vi "Histogram Main.vi"() -> ()   [LabVIEW 2014]
uses:
  Consumer Message.ctl
panel:
  out "Waveform Chart":dbl[](graph)=[-0.7333632170503996, -1.4459924395536827, -0.6158814268082136, -1.631675160365316, -1.608798951635636, -1.2625195714755832, -1.4388813392251412, -2.3171612936361585, -2.012658397448811, -2.452817845479024, -1.872742142198202, -1.8081370028145534, -2.789563597879967, -1.8027089686061069, -2.322157895514915, -2.6951322450543405, -2.70911241695026, -1.9297374709836919, -2.579302146161715, -2.341637191084045, -2.916687331127644, -2.8232178479366854, -2.1046997729908883, -2.788310680238794, -2.64060281585839, -2.904801503797829, -2.083598772555009, -2.2414412347815467, -2.3134391852883973, -2.2472652262621815, -2.459431080647101, -1.5756227831916778, -1.7057574382014546, -1.0977978414739988, -1.595566141630414, -1.0423098355592761, -1.5626121000032929, -0.9136565974827924, -1.1678232599898863, -1.0064070705532606, -0.34750263923649743, -0.46884042157229494, 0.0019576712199835256, -0.25029780993618395, 0.4362619199660559, 0.23147283969027768, 0.7382142888428814, 0.6139801858185563, 1.0184032107197016, 0.7597297806877022, 1.4420680686425897, 1.1325435146385732, 1.720696415405159, 1.2439523984726168, 1.7812438958662287, 1.4653663148145577, 2.2007124336943167, 1.8367478777079433, 1.5463773683452176, 2.5440750285679083, 2.354209943920518, 2.504065470614749, 1.6572648013533686, 2.746716411146539, 2.4693516941541107, 2.0377544919327506, 2.028659531799731, 2.373684202132056, 2.030316257851516, 1.9944781194585937, 3.0612841364650025, 2.459440160574936, 2.695378131255343, 1.88317869797155, 2.4020213090840583, 1.9296628462729055, 2.0296568601608906, 2.662724277929503, 2.3134823505056046, 1.9158567122932988, 2.1398584968764776, 1.540815181341315, 1.3225488335799052, 1.7322571649762133, 1.449096031199046, 1.1359472555523311, 0.7462838155083935, 1.4330296047378257, 1.3257675163227414, 0.7403863574684398, 0.8139573928818378, 0.4596137579857783, 0.1374905254078728, -0.32650307170817594, -0.005885944408503383, -0.3876385007753408, 0.17942583515161425, -0.7655530391627472, -0.2667260819539556, -0.5640795763406656]
  in  "Snapshot":bool
  out "Histogram":cluster{"histogram":dbl[], "x axis":dbl[]}(graph)
  out "Consumer Shutdown?":bool=TRUE
  in  "Stop":bool
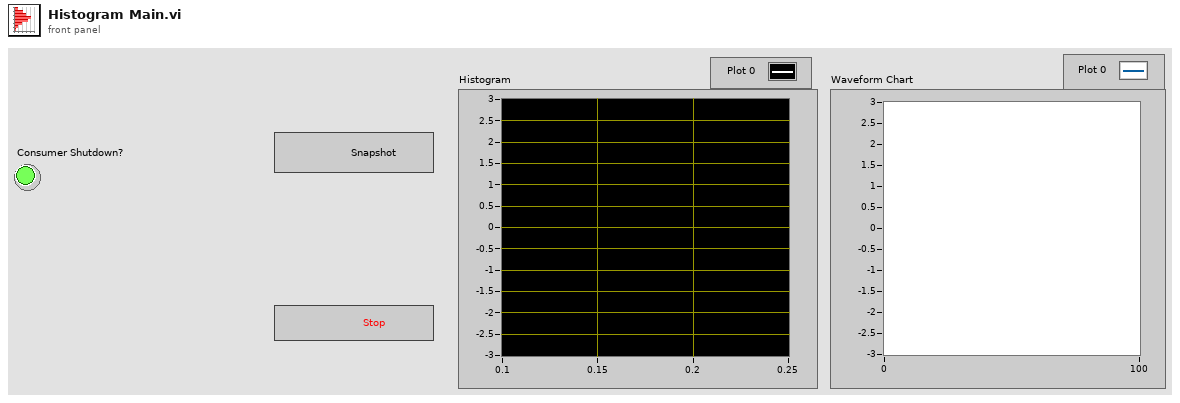
[diagram p1: front panel]
types:
  T1 = typedef "Consumer Message.ctl" = cluster{"Consumer State":string, "Boolean Data":bool, "Numeric Data":i32, "Signal":dbl[], "Error":errorcluster}
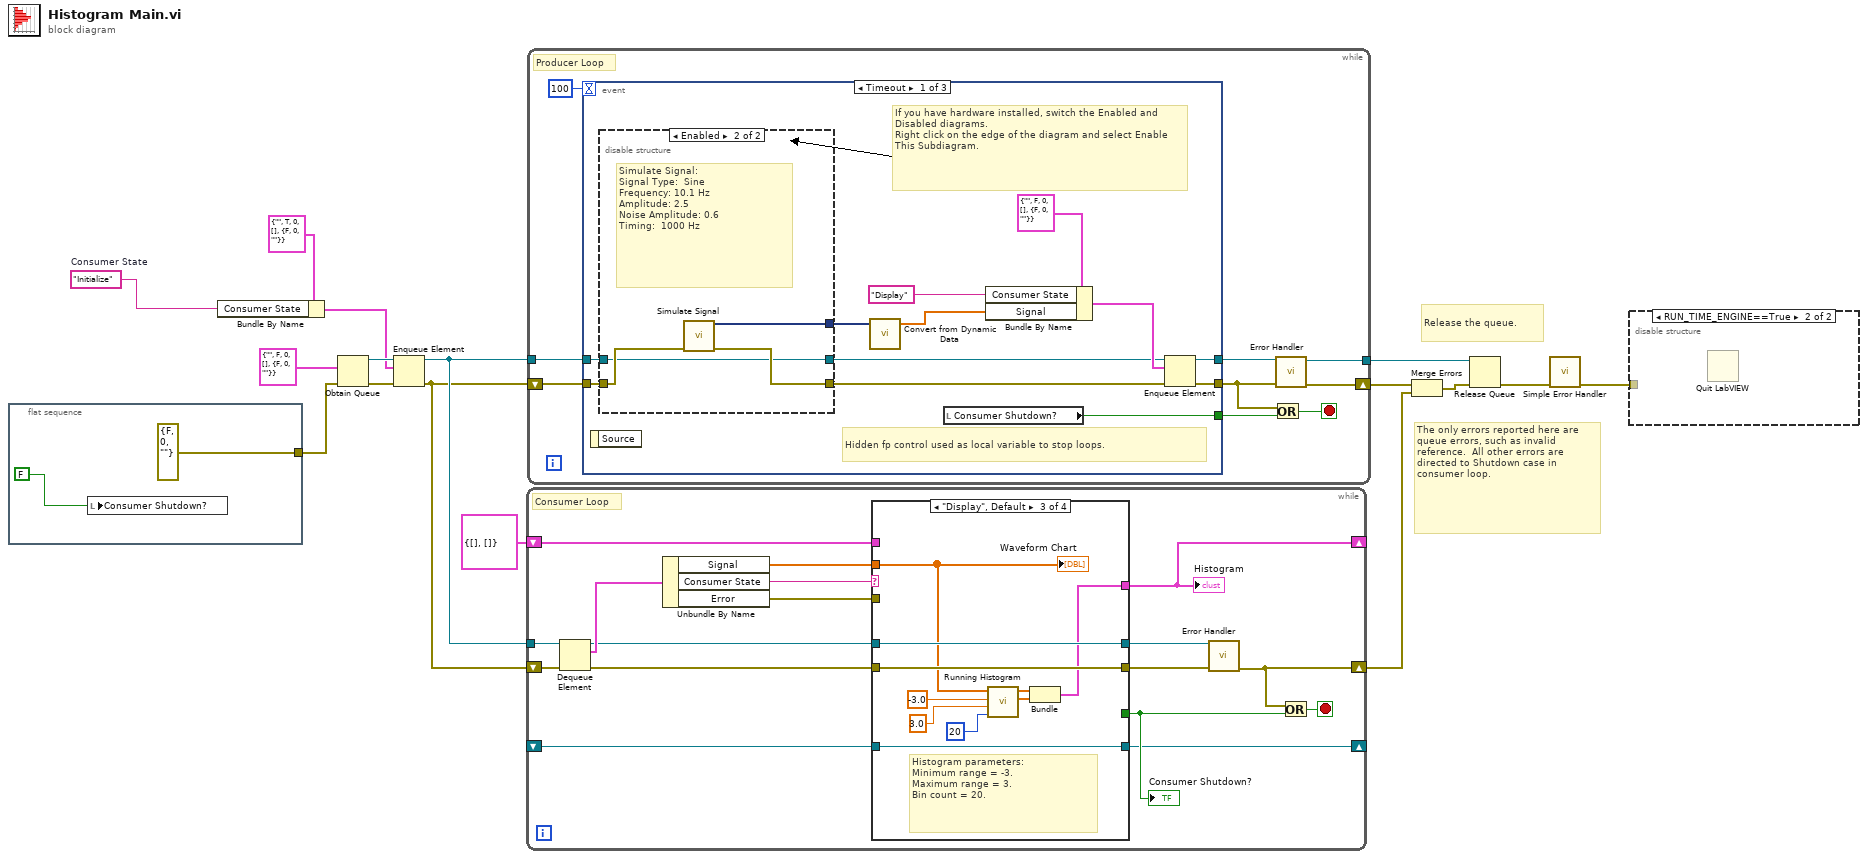
[diagram p0: block diagram]
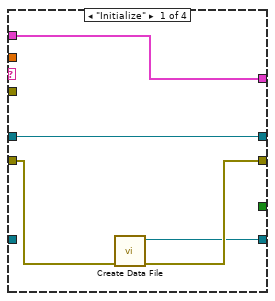
[diagram p3: hidden frame]
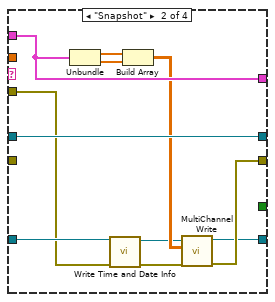
[diagram p4: hidden frame]
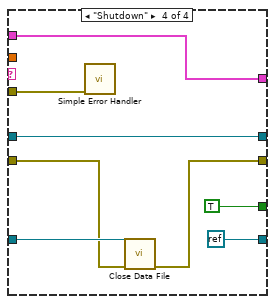
[diagram p5: hidden frame]
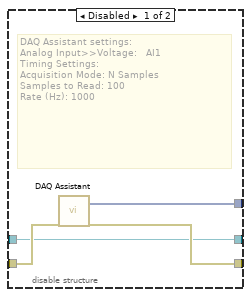
[diagram p6: hidden frame]
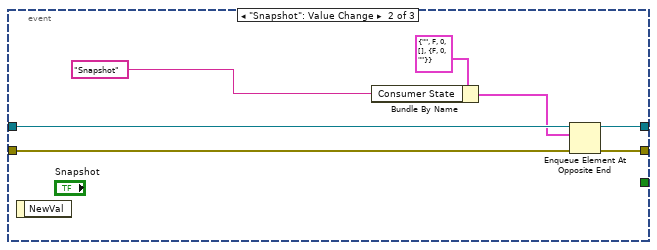
[diagram p7: hidden frame]
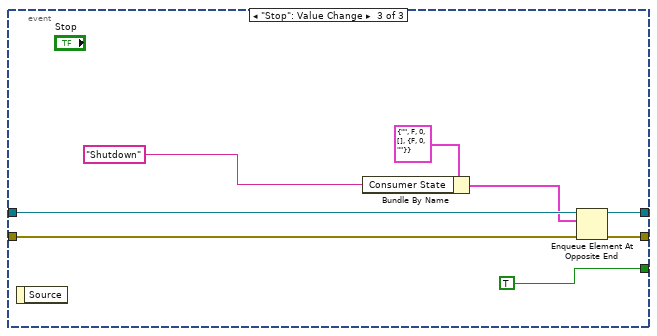
[diagram p8: hidden frame]
diagram:
  w9 = "Initialize"  # Consumer State
  # "Release the queue."
  # "The only errors reported here are queue errors, such as invalid reference.  All other errors are directed to Shutdown case in consumer loop."
  n1 = flat-sequence {
    tunnel: [errorcluster {"status"=FALSE, "code"=0, "source"=""} ("error in (no error)")] -> w12
    frame #0 {
      n2 = local write "Consumer Shutdown?"(FALSE ("Stop Loops (local)")) -> ()
    }
  }
  n3 = Bundle By Name(cluster=T1 {"Consumer State"="", "Boolean Data"=TRUE, "Numeric Data"=0, "Signal"=[], "Error"={"status"=FALSE, "code"=0, "source"=""}} ("Consumer Message"), "Consumer State"=w9) -> (w10:T1)
  n4 = Obtain Queue(element data type=T1 {"Consumer State"="", "Boolean Data"=FALSE, "Numeric Data"=0, "Signal"=[], "Error"={"status"=FALSE, "code"=0, "source"=""}}, error in (no error)=w12) -> (queue out=w14:refnum<queue>, error out=w16:errorcluster)  [unwired: 3 in, 1 out]
  n5 = Enqueue Element(queue=w14, element=w10, error in (no error)=w16) -> (queue out=w13:refnum<queue>, error out=w3:errorcluster)  [unwired: 1 in, 1 out]
  n6 = while {
    tunnel: w13 -> [w35]
    shift-right: [w26] -> w7
    shift-left: w3 -> [w34]
    shift-right: [w19] -> _
    shift-left: cluster{"histogram":dbl[], "x axis":dbl[]} {"histogram"=[], "x axis"=[]} -> [w23]
    shift-right: [w20] -> _
    shift-left: _ -> [w21]
    stop <- w27 stop-if-true
    # "Consumer Loop"
    n7 = Dequeue Element(queue=w35, error in (no error)=w34) -> (queue out=w25:refnum<queue>, element=w33:T1, error out=w24:errorcluster)  [unwired: 1 in, 1 out]
    n8 = Unbundle By Name(w33) -> ("Signal"=w22:dbl[], "Consumer State"=w32:string, "Error"=w29:errorcluster)
    n9 = case shown="\"Display\", Default" w32 {
      tunnel: [_ _ _ TRUE] -> w28
      tunnel: w24 -> [w38 _ w60 w64]
      tunnel: [w37 w47 w60 w63] -> w31
      tunnel: w25 -> [w40 w51 w61 w67]
      tunnel: [w40 w51 w61 w67] -> w30
      tunnel: w29 -> [_ w41 _ w68]
      tunnel: [w39 w49 w57 w66] -> w19
      tunnel: w23 -> [w39 w49 _ w66]
      tunnel: w22 -> [_ _ w55 _]
      tunnel: w21 -> [_ w42 w56 w65]
      tunnel: [w36 w46 w56 refnum<k0> refnum] -> w20
      frame "Initialize" {
        n10 = call "Create Data File.vi"("Error In"=w38) -> ("Error Out"=w37:errorcluster, "File Refnum"=w36:refnum<file>)  [unwired: 9 in]
      }
      frame "Snapshot" {
        n11 = Unbundle(w49) -> ("histogram"=w45:dbl[], "x axis"=w50:dbl[])
        n12 = call "Write Time and Date Info.vi"("Error In"=w41, "File Refnum In"=w42) -> ("Error Out"=w43:errorcluster, "File Refnum Out"=w44:refnum<file>)  [unwired: 6 in]
        n13 = Build Array(w45, w50) -> (w48:dbl[][])
        n14 = call "MultiChannel Write.vi"("Error In"=w43, "Data to Log"=w48, "File Refnum In"=w44) -> ("Error Out"=w47:errorcluster, "File Refnum Out"=w46:refnum<file>)  [unwired: 7 in]
      }
      frame "Display", Default {
        # "Histogram parameters:\nMinimum range = -3.\nMaximum range = 3. \nBin count = 20."
        n15 = call "Running Histogram.vi"("bins"=20, "max"=3.0, "min"=-3.0, "input data"=w55) -> ("x axis"=w58:dbl[], "histogram"=w59:dbl[])  [unwired: 4 in, 2 out]
        n16 = Bundle("histogram"=w59, "x axis"=w58) -> (w57:cluster{"histogram":dbl[], "x axis":dbl[]})  [unwired: 1 in]
        "Waveform Chart" <- w55
      }
      frame "Shutdown" {
        n17 = call <vilib>:"Simple Error Handler.vi"("error in (no error)"=w68) -> ()  [unwired: 4 in, 5 out]
        n18 = call "Close Data File.vi"("error in"=w64, "File Refnum In"=w65) -> ("error out"=w63:errorcluster)  [unwired: 9 in]
      }
    }
    "Consumer Shutdown?" <- w28
    "Histogram" <- w19
    n19 = call "Error Handler.vi"("error in"=w31, "queue in"=w30) -> ("error out"=w26:errorcluster)  [unwired: 8 in, 1 out]
    n20 = Or(x=w26, y=w28) -> (x .or. y?=w27:bool)
  }
  n21 = while {
    tunnel: w13 -> [w78]
    shift-right: [w71] -> w8
    shift-left: w3 -> [w77]
    tunnel: [w70] -> w2
    stop <- w73 stop-if-true
    # "Producer Loop"
    n22 = event shown="[0] Timeout" {
      selector: _ -> [_ _ _]
      dyn-events: _ -> [_ _ _]
      timeout: 100 -> [_ _ _]
      tunnel: w78 -> [w80 w104 w113]
      tunnel: w77 -> [w82 w103 w111]
      tunnel: [w85 w105 w110] -> w72
      tunnel: [w90 _ TRUE] -> w74
      tunnel: [w86 w100 w109] -> w76
      event Timeout {
        # "If you have hardware installed, switch the Enabled and Disabled diagrams.\nRight click on the edge of the diagram and select Enable This Subdiagram."
        # "Hidden fp control used as local variable to stop loops."
        n23 = event-data() -> ()  [unwired: 1 in, 1 out]
        n24 = disable-structure shown="Enabled" {
          disable-tunnel: [w94 w96] -> w83
          disable-tunnel: w82 -> [w93 w98]
          disable-tunnel: [w92 w97] -> w81
          disable-tunnel: w80 -> [w91 w95]
          disable-tunnel: [w91 w95] -> w79
          frame Disabled {
            # "DAQ Assistant settings:\nAnalog Input>>Voltage:   AI1\nTiming Settings:\nAcquisition Mode: N Samples\nSamples to Read: 100\nRate (Hz): 1000"
            n25 = call "DAQ Assistant"("error in"=w93) -> ("data"=w94:dynamicdata, "error out"=w92:errorcluster)  [unwired: 16 in, 1 out]
          }
          frame Enabled {
            # "Simulate Signal:\nSignal Type:  Sine\nFrequency: 10.1 Hz\nAmplitude: 2.5\nNoise Amplitude: 0.6\nTiming:  1000 Hz"
            n26 = call "Simulate Signal"("error in (no error)"=w98) -> ("Sine with Uniform Noise"=w96:dynamicdata, "error out"=w97:errorcluster)  [unwired: 13 in]
          }
        }
        n27 = call "Convert from Dynamic Data"("Dynamic Data Type"=w83) -> ("Array"=w84:dbl[])  [unwired: 3 in]
        n28 = local read "Consumer Shutdown?"() -> (w90:bool)
        n29 = Bundle By Name(cluster=T1 {"Consumer State"="", "Boolean Data"=FALSE, "Numeric Data"=0, "Signal"=[], "Error"={"status"=FALSE, "code"=0, "source"=""}}, "Consumer State"="Display", "Signal"=w84) -> (w88:T1)
        n30 = Enqueue Element(queue=w79, element=w88, error in (no error)=w81) -> (queue out=w86:refnum<queue>, error out=w85:errorcluster)  [unwired: 1 in, 1 out]
      }
      event "Snapshot": Value Change {
        n31 = event-data() -> ()  [unwired: 1 in, 1 out]
        n32 = Bundle By Name(cluster=T1 {"Consumer State"="", "Boolean Data"=FALSE, "Numeric Data"=0, "Signal"=[], "Error"={"status"=FALSE, "code"=0, "source"=""}}, "Consumer State"="Snapshot" ("String Data")) -> (w101:T1)
        n33 = Enqueue Element At Opposite End(queue=w104, element=w101, error in (no error)=w103) -> (queue out=w100:refnum<queue>, error out=w105:errorcluster)  [unwired: 1 in, 1 out]
      }
      event "Stop": Value Change {
        n34 = event-data() -> ()  [unwired: 1 in, 1 out]
        n35 = Bundle By Name(cluster=T1 {"Consumer State"="", "Boolean Data"=FALSE, "Numeric Data"=0, "Signal"=[], "Error"={"status"=FALSE, "code"=0, "source"=""}}, "Consumer State"="Shutdown") -> (w106:T1)
        n36 = Enqueue Element At Opposite End(queue=w113, element=w106, error in (no error)=w111) -> (queue out=w109:refnum<queue>, error out=w110:errorcluster)  [unwired: 1 in, 1 out]
      }
    }
    n37 = Or(x=w72, y=w74) -> (x .or. y?=w73:bool)
    n38 = call "Error Handler.vi"("error in"=w72, "queue in"=w76) -> ("error out"=w71:errorcluster, "queue out"=w70:refnum<queue>)  [unwired: 8 in]
  }
  n39 = Merge Errors(w8, w7) -> (w5:errorcluster)
  n40 = Release Queue(queue=w2, error in (no error)=w5) -> (error out=w4:errorcluster)  [unwired: 1 in, 2 out]
  n41 = call <vilib>:"Simple Error Handler.vi"("error in (no error)"=w4) -> ("error out"=w1:errorcluster)  [unwired: 4 in, 4 out]
  n42 = disable-structure shown="RUN_TIME_ENGINE==True" {
    disable-tunnel: w1 -> [_ _]
    frame condition #0 (active) {
    }
    frame condition #1 {
      n43 = Quit LabVIEW() -> ()  [unwired: 1 in]
    }
  }
